vi "calcUk.vi"(8 "error in (no error)":errorcluster, 9 "dofIdx":i32[](array[numeric]), 10 "Qx Array":dbl[][](array[numeric]), 11 "OptCtrl in":refnum<class "OptCtrl.lvclass">) -> (0 "error out":errorcluster, 2 "uk Array":dbl[](array[numeric]), 3 "OptCtrl out":refnum<class "OptCtrl.lvclass">)   [LabVIEW 2016, in "OptCtrl.lvclass"]
doc: "Calculate uk by referencing to \"0\", \"x0\", or \"x00\" based on the configuration file."
uses:
  OptCtrl.lvclass
  OptCtrl.lvclass/OptCtrl.ctl
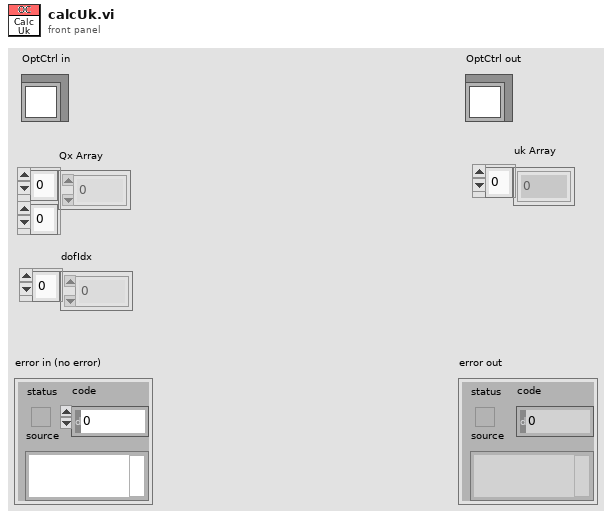
[diagram p1: front panel]
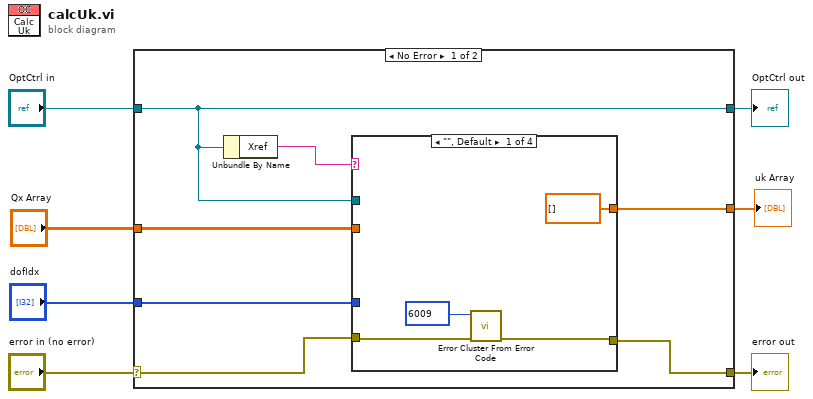
[diagram p0: block diagram]
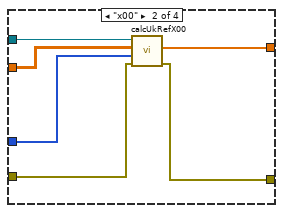
[diagram p2: hidden frame]
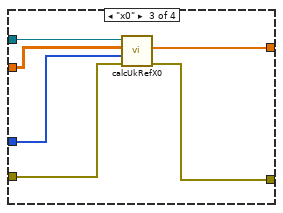
[diagram p3: hidden frame]
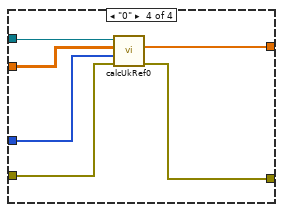
[diagram p4: hidden frame]
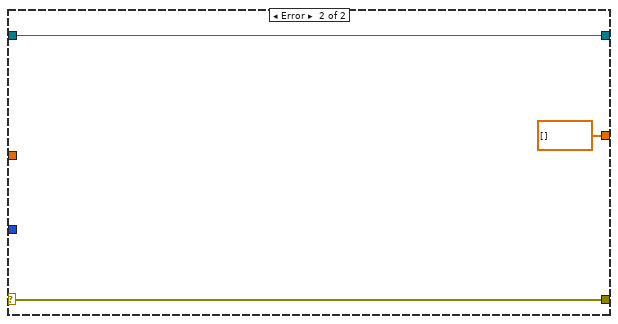
[diagram p5: hidden frame]
diagram:
  n1 = case shown="No Error" "error in (no error)" {
    selector: "error in (no error)" -> [w9 w39]
    tunnel: [w8 w39] -> w6
    tunnel: [w11 w38] -> w4
    tunnel: "OptCtrl in" -> [w11 w38]
    tunnel: "Qx Array" -> [w13 _]
    tunnel: "dofIdx" -> [w12 _]
    tunnel: [w10 dbl[] [] ("uk Array")] -> w1
    frame No Error {
      n2 = Unbundle By Name(w11) -> ("Xref"=w14:string)
      n3 = case shown="\"\", Default" w14 {
        tunnel: w13 -> [_ w23 w29 w35]
        tunnel: w12 -> [_ w22 w28 w34]
        tunnel: w11 -> [_ w24 w30 w36]
        tunnel: [dbl[] [] ("uk Array") w21 w25 w31] -> w10
        tunnel: w9 -> [w16 w20 w27 w33]
        tunnel: [w15 w19 w26 w32] -> w8
        frame "", Default {
          n4 = call <vilib>:"Error Cluster From Error Code.vi"("error in (no error)"=w16, "error code (0)"=6009 ("code")) -> ("error out"=w15:errorcluster)  [unwired: 7 in]
        }
        frame "x00" {
          n5 = call "calcUkRefX00.vi"("error in (no error)"=w20, "dofIdx"=w22, "Qx Array"=w23, "OptCtrl in"=w24) -> ("error out"=w19:errorcluster, "uk Array"=w21:dbl[])  [unwired: 5 in, 1 out]
        }
        frame "x0" {
          n6 = call "calcUkRefX0.vi"("error in (no error)"=w27, "dofIdx"=w28, "Qx Array"=w29, "OptCtrl in"=w30) -> ("error out"=w26:errorcluster, "uk Array"=w25:dbl[])  [unwired: 5 in, 1 out]
        }
        frame "0" {
          n7 = call "calcUkRef0.vi"("error in (no error)"=w33, "dofIdx"=w34, "Qx Array"=w35, "OptCtrl in"=w36) -> ("error out"=w32:errorcluster, "uk Array"=w31:dbl[])  [unwired: 5 in, 1 out]
        }
      }
    }
    frame Error {
    }
  }
  "error out" <- w6
  "OptCtrl out" <- w4
  "uk Array" <- w1
